vi "Create DoubleArrayMsg.vi"(8 "error in (no error)":errorcluster, 10 "Message Data":dbl[](array[numeric]), 11 "Message Name":string) -> (0 "error out":errorcluster, 3 "DoubleArrayMsg Out":refnum<class "DoubleArrayMsg.lvclass">)   [LabVIEW 2018, in "LapDog.Messaging.v3.NativeArrays.lvlib" / "DoubleArrayMsg.lvclass"]
doc: "Returns a DoubleArrayMsg object with the given name.\n\nThis method executes regardless of the error in state."
uses:
  DoubleArrayMsg.lvclass
  T:/git/LapDog.Messaging/src/LapDog.Messaging/Message/Message.lvclass
  DoubleArrayMsg.lvclass/DoubleArrayMsg.ctl
  LapDog.Messaging/Message/Message.lvclass
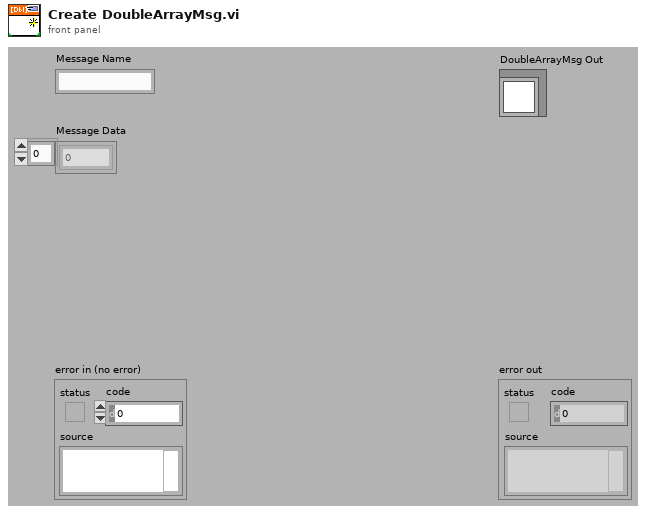
[diagram p1: front panel]
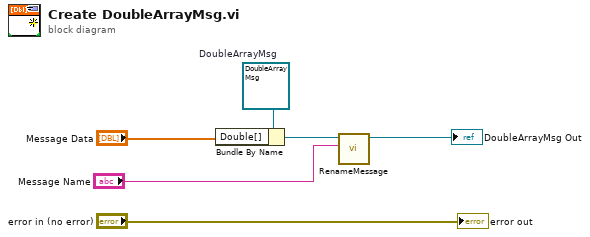
[diagram p0: block diagram]
diagram:
  w6 = refnum<class "DoubleArrayMsg.lvclass"> refnum  # DoubleArrayMsg
  n1 = Bundle By Name(cluster=w6, "Double[]"="Message Data") -> (w3:refnum<class "DoubleArrayMsg.lvclass">)
  n2 = call "RenameMessage.vi"("Message Name"="Message Name", "Message in"=w3) -> ("Message out"=→"DoubleArrayMsg Out":refnum<class "DoubleArrayMsg.lvclass">)  [unwired: 8 in, 1 out]
  "error out" <- "error in (no error)"
